vi "InitFourStack.vi"(8 "Fourth":refnum<class "ActionStack.lvclass">, 9 "Third":refnum<class "ActionStack.lvclass">, 10 "Second":refnum<class "ActionStack.lvclass">, 11 "ActionStack in":refnum<class "ActionStack.lvclass">) -> (1 "Actions":refnum<class "ActionStack.lvclass">[](array[class]))   [LabVIEW 2024]
uses:
  ActionStack.lvclass
  ActionStack.lvclass/ActionStack.ctl
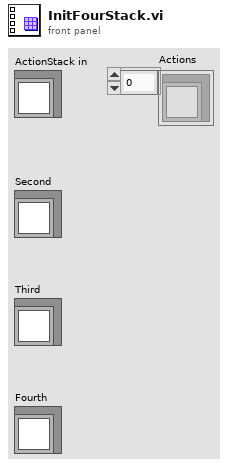
[diagram p1: front panel]
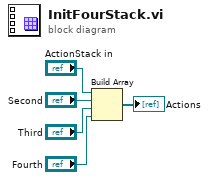
[diagram p0: block diagram]
diagram:
  n1 = Build Array("ActionStack in", "Second", "Third", "Fourth") -> (→"Actions":refnum<class "ActionStack.lvclass">[])
